vi "Wiimote Get Core Buttons.vi"(8 "error in":errorcluster, 11 "hWiimoteHandle in":u32 format="%08x") -> (0 "error out":errorcluster, 2 "Wiimote Buttons out":T1, 3 "hWiimoteHandle out":u32 format="%08x")   [LabVIEW 2011, in "Wiimote.lvlib"]
uses:
  Wiimote.lvlib
  Wiimote Buttons.ctl
  Wiimote Reporting Mode.ctl
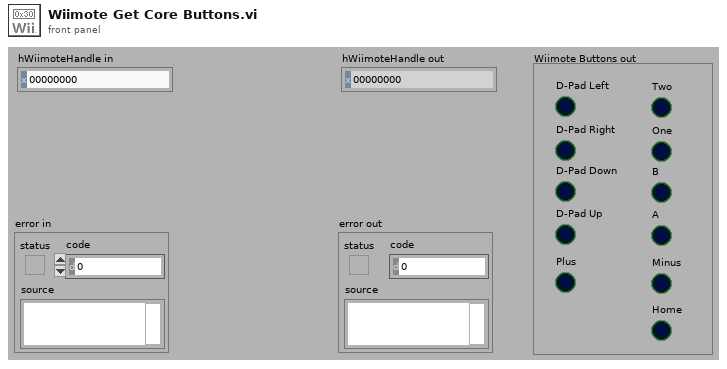
[diagram p1: front panel]
types:
  T1 = typedef "Wiimote.lvlib/Wiimote Buttons.ctl" = cluster{"D-Pad Left":bool, "D-Pad Right":bool, "D-Pad Down":bool, "D-Pad Up":bool, "Plus":bool, "Two":bool, "One":bool, "B":bool, "A":bool, "Minus":bool, "Home":bool}
  T2 = typedef "Wiimote.lvlib/Wiimote Reporting Mode.ctl" = u8
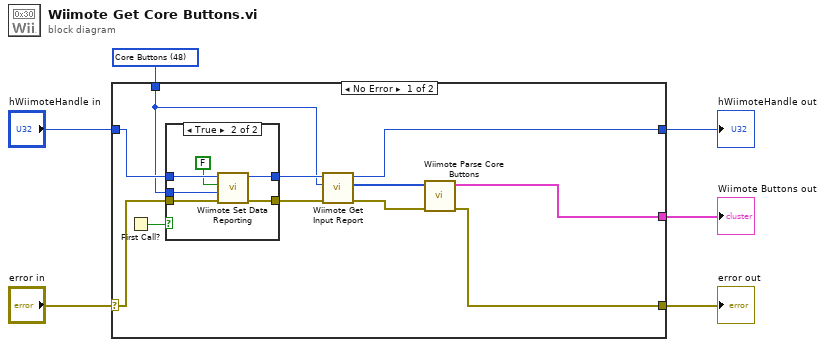
[diagram p0: block diagram]
diagram:
  w1 = T2 48 items=["Core Buttons"=48, "Core Buttons and Accelerometer"=49, "Core Buttons with 8 Extension bytes"=50, "Core Buttons and Accelerometer with 12 IR bytes"=51, "Core Buttons with 19 Extension bytes"=52, "Core Buttons and Accelerometer with 16 Extension Bytes"=53, "Core Buttons with 10 IR bytes and 9 Extension Bytes"=54, "Core Buttons and Accelerometer with 10 IR bytes and 6 Extension Bytes"=55] ("Reporting Mode")
  n1 = case shown="No Error" "error in" {
    selector: "error in" -> [w9 w27]
    tunnel: [w16 w27] -> w5
    tunnel: "hWiimoteHandle in" -> [w10 w26]
    tunnel: [w15 w26] -> w3
    tunnel: [w13 _] -> w2
    tunnel: w1 -> [w7 _]
    frame No Error {
      n2 = First Call?() -> (First Call?: T/F=w11:bool)
      n3 = case shown="True" w11 {
        tunnel: [w19 w25] -> w12
        tunnel: w10 -> [w19 w24]
        tunnel: w9 -> [w18 w23]
        tunnel: [w18 w22] -> w8
        tunnel: w7 -> [_ w20]
        frame False {
        }
        frame True {
          n4 = call "Wiimote Set Data Reporting.vi"("error in"=w23, "Reporting Mode"=w20, "Continuous"=FALSE, "hWiimoteHandle in"=w24) -> ("error out"=w22:errorcluster, "hWiimoteHandle out"=w25:u32)  [unwired: 6 in]
        }
      }
      n5 = call "Wiimote Get Input Report.vi"("error in"=w8, "bInputReport"=w7, "hWiimoteHandle in"=w12) -> ("error out"=w17:errorcluster, "pReportBuffer out"=w14:u8[], "hWiimoteHandle out"=w15:u32)  [unwired: 6 in]
      n6 = call "Wiimote Parse Core Buttons.vi"("error in"=w17, "pReportBuffer in"=w14) -> ("error out"=w16:errorcluster, "Wiimote Buttons out"=w13:T1)  [unwired: 8 in]
    }
    frame Error {
    }
  }
  "error out" <- w5
  "hWiimoteHandle out" <- w3
  "Wiimote Buttons out" <- w2
